vi "lib bool to enable disable.vi"(10 "Boolean":bool) -> (2 "Enable/Disable":T1(ring))   [LabVIEW 2015]
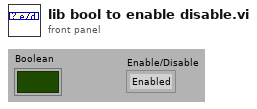
[diagram p1: front panel]
types:
  T1 = enum8{"Enabled", "Disabled", "Disabled and Grayed Out"}
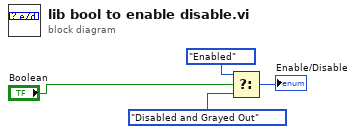
[diagram p0: block diagram]
diagram:
  n1 = Select(t=T1."Enabled" ("Disabled"), s="Boolean", f=T1."Disabled and Grayed Out" ("Disabled")) -> (s? t:f=→"Enable/Disable":T1)
